vi "(PART 1) Minimum and Maximum.vi"() -> ()   [LabVIEW 2015]
panel:
  out "?":dbl
  out "ITERRATION COUNT":dbl
  out "CURRENT MINIMUM":dbl
  out "CURRENT MAXIMUM":dbl
  # "CURRENT NUMBER"
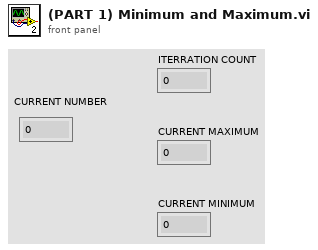
[diagram p1: front panel]
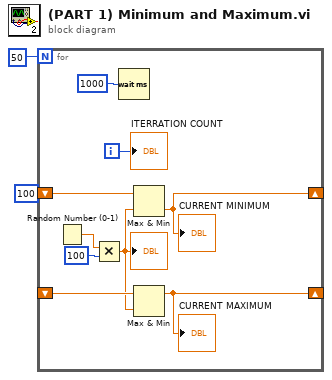
[diagram p0: block diagram]
diagram:
  n1 = for {
    N: 50 -> [_]
    shift-right: [w9] -> _
    shift-left: _ -> [w7]
    shift-right: [w8] -> _
    shift-left: 100 -> [w6]
    i -> [w10]
    n2 = Random Number (0-1)() -> (number: 0 to 1=w5:dbl)
    n3 = Multiply(x=w5, y=100) -> (x*y=w3:dbl)
    "?" <- w3
    n4 = Wait (ms)(milliseconds to wait=1000) -> ()  [unwired: 1 out]
    n5 = Max & Min(x=w6, y=w3) -> (min(x,y)=w8:dbl)  [unwired: 1 out]
    "CURRENT MINIMUM" <- w8
    n6 = Max & Min(x=w7, y=w3) -> (max(x,y)=w9:dbl)  [unwired: 1 out]
    "CURRENT MAXIMUM" <- w9
    "ITERRATION COUNT" <- w10
  }
